vi "DSF.Engine.Transceiver Thread.Rx.vi"(8 "error in (no error)":errorcluster, 10 "Transfer Group in":refnum<class "DSF.Engine.Transfer Group.lvclass">, 11 "Transceiver Thread in":refnum<class "DSF.Engine.Transceiver Thread.lvclass">) -> (0 "error out":errorcluster, 2 "Transfer Group out":refnum<class "DSF.Engine.Transfer Group.lvclass">, 3 "Transceiver Thread out":refnum<class "DSF.Engine.Transceiver Thread.lvclass">)   [LabVIEW 2017, in "Data Sharing Framework Engine.lvlib" / "DSF.Engine.Transceiver Thread.lvclass"]
uses:
  DSF.Engine.Transceiver Thread.lvclass
  Transfer/DSF.Engine.Transfer Group.lvclass
  DSF.Engine.Transceiver Thread.lvclass/DSF.Engine.Transceiver Thread.ctl
  DSF.Engine.Transceiver.lvclass
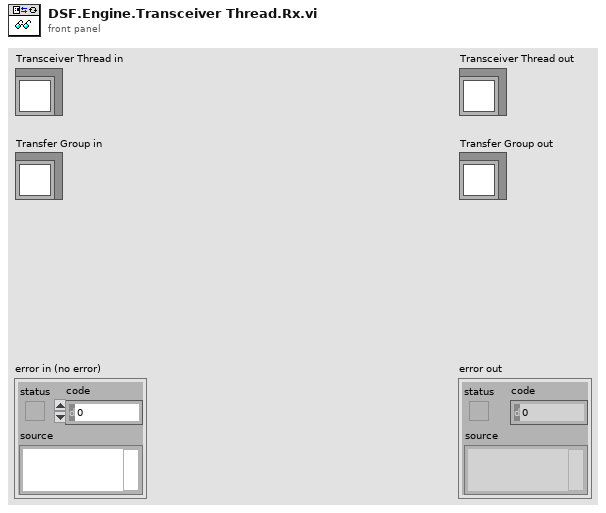
[diagram p1: front panel]
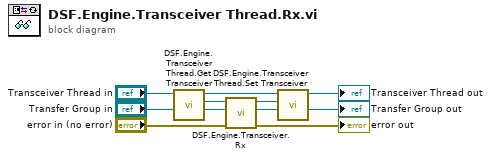
[diagram p0: block diagram]
diagram:
  n1 = call "DSF.Engine.Transceiver Thread.Get Transceiver.vi"("Transceiver Thread in"="Transceiver Thread in") -> ("Transceiver"=w9:refnum<class "DSF.Engine.Transceiver.lvclass">, "Transceiver Thread out"=w7:refnum<class "DSF.Engine.Transceiver Thread.lvclass">)  [unwired: 9 in]
  n2 = call-dynamic "DSF.Engine.Transceiver.Rx.vi"("error in (no error)"="error in (no error)", "Transfer Group in"="Transfer Group in", "Transceiver in"=w9) -> ("error out"=→"error out":errorcluster, "Transfer Group out"=→"Transfer Group out":refnum<class "DSF.Engine.Transfer Group.lvclass">, "Transceiver out"=w8:refnum<class "DSF.Engine.Transceiver.lvclass">)  [unwired: 6 in]
  n3 = call "DSF.Engine.Transceiver Thread.Set Transceiver.vi"("Transceiver"=w8, "Transceiver Thread in"=w7) -> ("Transceiver Thread out"=→"Transceiver Thread out":refnum<class "DSF.Engine.Transceiver Thread.lvclass">)  [unwired: 9 in]
